vi "Shoot.vi"(8 "Reset":bool, 11 "Shooter Sensor":bool) -> (0 "Arm fingers state":T1, 1 "Finished?":bool, 2 "Roller Motor Value":dbl, 3 "Shooter Motor Value":dbl)   [LabVIEW 2013]
uses:
  <vilib>/Rock Robotics/WPI/Solenoid/WPI_SolenoidValue.ctl
  Shoot States.ctl
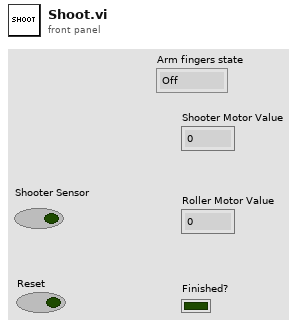
[diagram p1: front panel]
types:
  T1 = typedef "WPI_SolenoidValue.ctl" = enum16{"Off", "On", "Forward", "Reverse"}
  T2 = typedef "Shoot States.ctl" = enum16{"Get time", "Wait for False", "Wait for True", "Finished", "Open Fingers", "Close Fingers"}
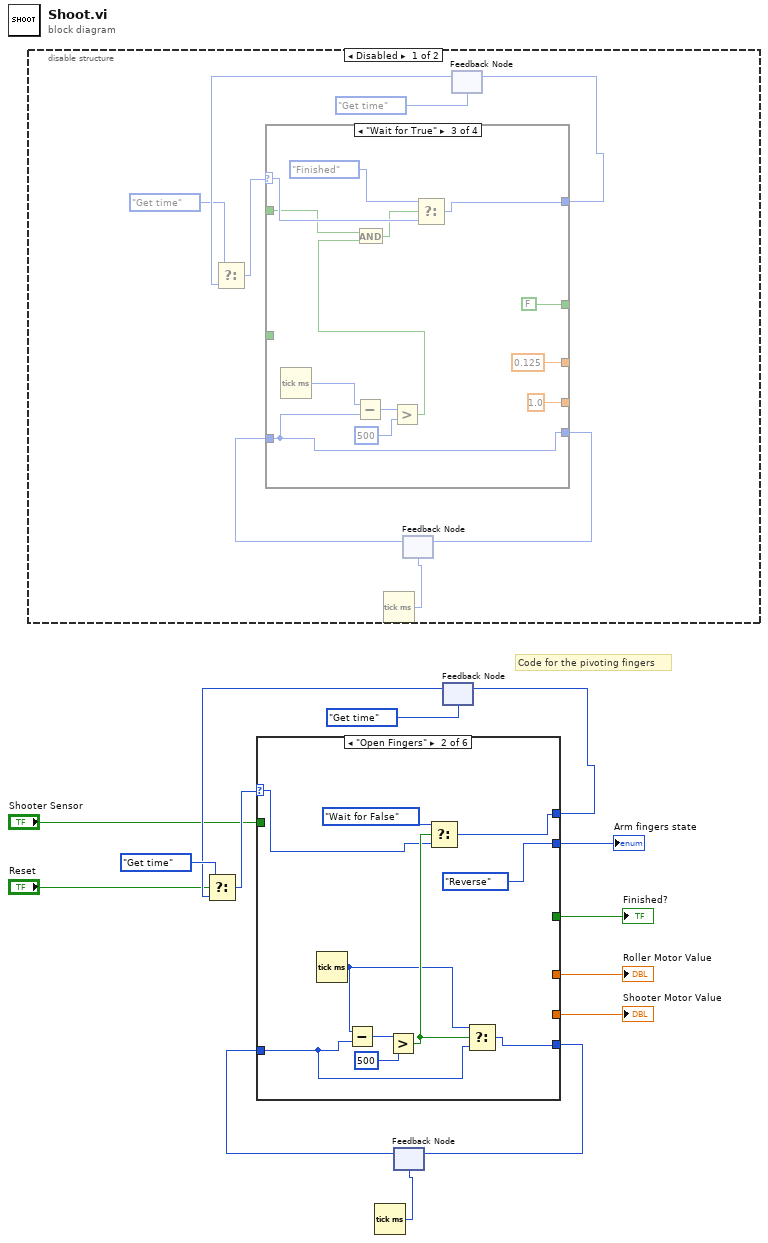
[diagram p0: block diagram]
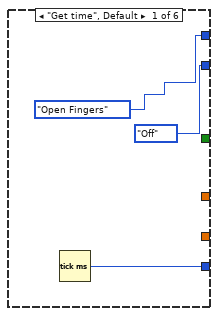
[diagram p2: hidden frame]
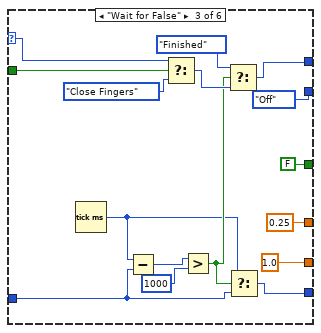
[diagram p3: hidden frame]
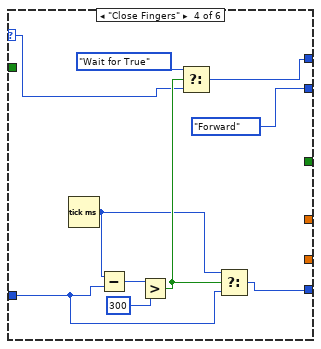
[diagram p4: hidden frame]
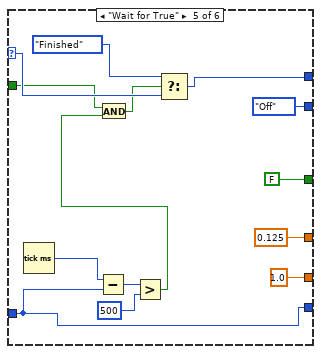
[diagram p5: hidden frame]
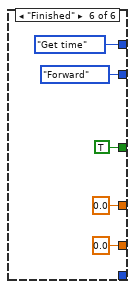
[diagram p6: hidden frame]
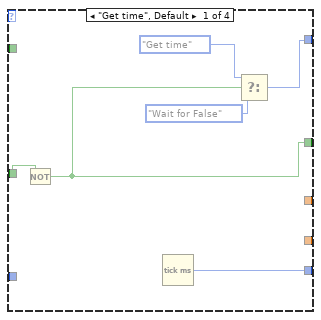
[diagram p7: hidden frame]
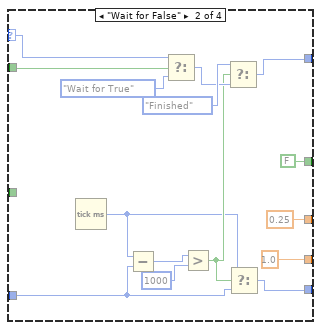
[diagram p8: hidden frame]
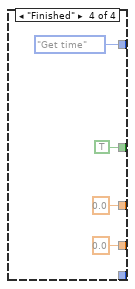
[diagram p9: hidden frame]
diagram:
  # "Code for the pivoting fingers"
  n1 = disable-structure shown="Disabled" {
    frame Disabled {
      n2 = Tick Count (ms)() -> (millisecond timer value=w15:u32)
      n3 = feedback #1(w15) -> (w22:u32)
      n4 = feedback #2(Shoot_States."Get time") -> (w19:T2)
      n5 = Select(t=Shoot_States."Get time", f=w19) -> (s=w20:bool, s? t:f=w17:T2)
      n6 = case shown="\"Wait for True\"" w17 {
        selector: w17 -> [_ w44 w59 _]
        tunnel: [_ 0.25 0.125 0.0] -> _
        tunnel: [_ 1.0 1.0 0.0] -> _
        tunnel: [_ w41 w53 _] -> w24
        tunnel: [w29 FALSE FALSE TRUE] -> _
        tunnel: w22 -> [_ w33 w48 _]
        tunnel: [w31 w32 w48 _] -> w23
        tunnel: [w26 w37 w54 Shoot_States."Get time"] -> w21
        tunnel: [w30 _ _ _] -> w16
        frame "Get time", Default {
          n7 = Not(x=w30) -> (.not. x?=w29:bool)
          n8 = Tick Count (ms)() -> (millisecond timer value=w31:u32)
          n9 = Select(t=Shoot_States."Get time", s=w29, f=Shoot_States."Wait for False") -> (s? t:f=w26:T2)
        }
        frame "Wait for False" {
          n10 = Tick Count (ms)() -> (millisecond timer value=w34:u32)
          n11 = Subtract(x=w34, y=w33) -> (x-y=w43:u32)
          n12 = Select(t=w44, s=w41, f=Shoot_States."Wait for True") -> (s? t:f=w38:T2)
          n13 = Greater?(x=w43, y=u32 1000) -> (0:w35:bool)
          n14 = Select(t=Shoot_States."Finished" ("f"), s=w35, f=w38) -> (s? t:f=w37:T2)
          n15 = Select(t=w34, s=w35, f=w33) -> (s? t:f=w32:u32)
        }
        frame "Wait for True" {
          n16 = Tick Count (ms)() -> (millisecond timer value=w51:u32)
          n17 = Subtract(x=w51, y=w48) -> (x-y=w50:u32)
          n18 = Greater?(x=w50, y=u32 500) -> (0:w47:bool)
          n19 = And(x=w53, y=w47) -> (x .and. y?=w52:bool)
          n20 = Select(t=Shoot_States."Finished", s=w52, f=w59) -> (s? t:f=w54:T2)
        }
        frame "Finished" {
        }
      }
      n21 = feedback-in #1(w23) -> ()
      n22 = feedback-in #2(w21) -> ()
    }
    frame Enabled {
    }
  }
  n23 = Tick Count (ms)() -> (millisecond timer value=w14:u32)
  n24 = feedback #3(w14) -> (w9:u32)
  n25 = feedback #4(Shoot_States."Get time") -> (w11:T2)
  n26 = Select(t=Shoot_States."Get time", s="Reset", f=w11) -> (s? t:f=w13:T2)
  n27 = case shown="\"Open Fingers\"" w13 {
    selector: w13 -> [_ w67 w90 w93 w116 _]
    tunnel: [_ _ 0.25 _ 0.125 0.0] -> w4
    tunnel: [_ _ 1.0 _ 1.0 0.0] -> w5
    tunnel: "Shooter Sensor" -> [_ _ w87 _ w110 _]
    tunnel: [_ _ FALSE _ FALSE TRUE] -> w3
    tunnel: w9 -> [_ w69 w79 w95 w105 _]
    tunnel: [w66 w71 w78 w97 w105 _] -> w8
    tunnel: [Shoot_States."Open Fingers" w68 w83 w94 w111 Shoot_States."Get time"] -> w10
    tunnel: [WPI_SolenoidValue."Off" ("Arm Out") WPI_SolenoidValue."Reverse" ("Arm Out") WPI_SolenoidValue."Off" ("Arm Out") WPI_SolenoidValue."Forward" ("Arm Out") WPI_SolenoidValue."Off" ("Arm Out") WPI_SolenoidValue."Forward" ("Arm Out")] -> w6
    frame "Get time", Default {
      n28 = Tick Count (ms)() -> (millisecond timer value=w66:u32)
    }
    frame "Open Fingers" {
      n29 = Tick Count (ms)() -> (millisecond timer value=w70:u32)
      n30 = Subtract(x=w70, y=w69) -> (x-y=w75:u32)
      n31 = Greater?(x=w75, y=u32 500) -> (0:w72:bool)
      n32 = Select(t=Shoot_States."Wait for False", s=w72, f=w67) -> (s? t:f=w68:T2)
      n33 = Select(t=w70, s=w72, f=w69) -> (s? t:f=w71:u32)
    }
    frame "Wait for False" {
      n34 = Tick Count (ms)() -> (millisecond timer value=w80:u32)
      n35 = Subtract(x=w80, y=w79) -> (x-y=w89:u32)
      n36 = Select(t=w90, s=w87, f=Shoot_States."Close Fingers") -> (s? t:f=w84:T2)
      n37 = Greater?(x=w89, y=u32 1000) -> (0:w81:bool)
      n38 = Select(t=Shoot_States."Finished" ("f"), s=w81, f=w84) -> (s? t:f=w83:T2)
      n39 = Select(t=w80, s=w81, f=w79) -> (s? t:f=w78:u32)
    }
    frame "Close Fingers" {
      n40 = Tick Count (ms)() -> (millisecond timer value=w96:u32)
      n41 = Subtract(x=w96, y=w95) -> (x-y=w101:u32)
      n42 = Greater?(x=w101, y=u32 300) -> (0:w98:bool)
      n43 = Select(t=Shoot_States."Wait for True", s=w98, f=w93) -> (s? t:f=w94:T2)
      n44 = Select(t=w96, s=w98, f=w95) -> (s? t:f=w97:u32)
    }
    frame "Wait for True" {
      n45 = Tick Count (ms)() -> (millisecond timer value=w108:u32)
      n46 = Subtract(x=w108, y=w105) -> (x-y=w107:u32)
      n47 = Greater?(x=w107, y=u32 500) -> (0:w104:bool)
      n48 = And(x=w110, y=w104) -> (x .and. y?=w109:bool)
      n49 = Select(t=Shoot_States."Finished", s=w109, f=w116) -> (s? t:f=w111:T2)
    }
    frame "Finished" {
    }
  }
  "Arm fingers state" <- w6
  "Shooter Motor Value" <- w5
  "Finished?" <- w3
  "Roller Motor Value" <- w4
  n50 = feedback-in #3(w8) -> ()
  n51 = feedback-in #4(w10) -> ()
